vi "Q_Insert VI By Ref.vi"(8 "error in":errorcluster caption="错误输入（无错误）", 10 "Dynamic VI*":refnum<vi>, 11 "ChildNode*":refnum<data-value>) -> (0 "error out":errorcluster caption="错误输出")   [LabVIEW 2016, in "PanelDataNode.lvclass"]
uses:
  PanelDataNode.lvclass
  PanelDataNode.lvclass/PanelDataNode.ctl
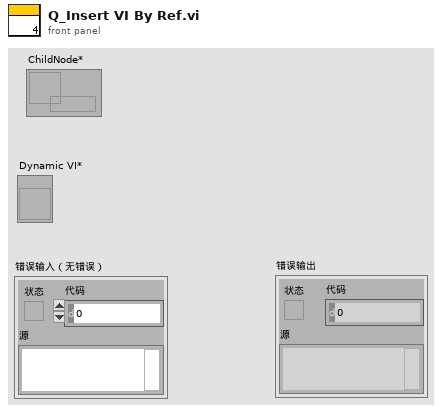
[diagram p1: front panel]
types:
  T1 = cluster{"ChildNode*":refnum<data-value>, "Dynamic VI*":refnum<vi>}
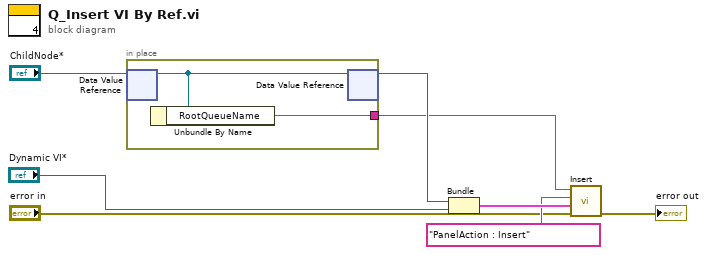
[diagram p0: block diagram]
diagram:
  n1 = in-place {
    in-place-border: [w10] -> w4
    n2 = in-place-dvr #1("ChildNode*") -> (w9:refnum<class "PanelDataNode.lvclass">)  [unwired: 1 out]
    n3 = Unbundle By Name(w9) -> ("RootQueueName"=w10:string)
    n4 = in-place-dvr #1(w9) -> (w5:refnum<data-value>)  [unwired: 1 out]
  }
  n5 = Bundle("ChildNode*"=w5, "Dynamic VI*"="Dynamic VI*") -> (w8:T1)  [unwired: 1 in]
  n6 = call "Insert.vi"("error in"="error in", "Data"=w8, "Event"="PanelAction : Insert", "QueueName"=w4) -> ("error out"=→"error out":errorcluster)  [unwired: 6 in, 1 out]
